vi "File Run.vi"(7 "Write Period":u32=3000, 8 "Error In":errorcluster) -> (0 "Error Out":errorcluster)   [LabVIEW 2017, in "Logger.lvlib"]
doc: "Continuously writes logging statements to the default log file. This VI is called by the File State VI in the background, but if background operation is disabled, then this VI needs to be explicitly placed in the block diagram of the top level application VI."
uses:
  Logger.lvlib
  Private/Control Action.ctl
  Private/File/Action.ctl
  Private/File/File.lvlib
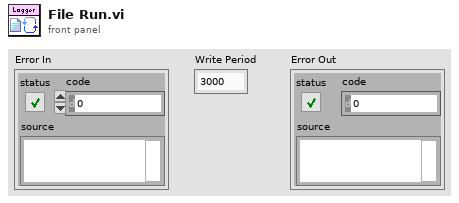
[diagram p1: front panel]
types:
  T1 = typedef "Logger.lvlib/Control Action.ctl" = enum16{"Initialize", "Get", "Set", "Shutdown"}
  T2 = typedef "Logger.lvlib/File.lvlib/Action.ctl" = enum16{"Initialize", "Set Maximum File Size", "Set Maximum File Count", "Set Root Folder", "Set Enable Calendar Folder Tree", "Set File Extension", "Start", "Write", "Stop", "Shutdown"}
  T3 = typedef "Logger.lvlib/Statement.ctl" = cluster{"Time Stamp":timestamp, "Tag":T4, "Source":string, "Message":string}
  T4 = typedef "Logger.lvlib/Tag.ctl" = enum16{"Fatal", "Error", "Warn", "Info", "Debug", "Trace"}
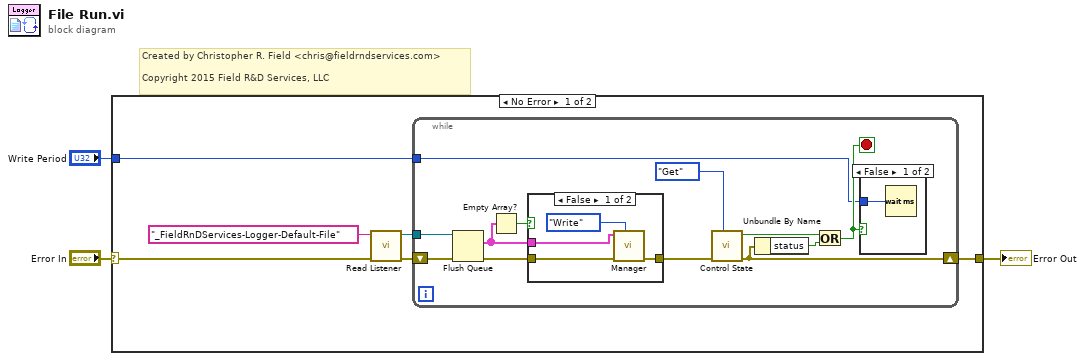
[diagram p0: block diagram]
diagram:
  # "Created by Christopher R. Field <chris@fieldrndservices.com>\n\nCopyright 2015 Field R&D Services, LLC"
  n1 = case shown="No Error" "Error In" {
    selector: "Error In" -> [w9 w28]
    tunnel: [w6 w28] -> w2
    tunnel: "Write Period" -> [w4 _]
    frame No Error {
      n2 = call "Read Listener.vi"("Error In"=w9, "Listener ID"="_FieldRnDServices-Logger-Default-File") -> ("Error Out"=w7:errorcluster, "Listener"=w8:refnum<queue>)  [unwired: 8 in]
      n3 = while {
        tunnel: w8 -> [w21]
        shift-right: [w11] -> w6
        shift-left: w7 -> [w20]
        tunnel: w4 -> [w10]
        stop <- w12 stop-if-true
        n4 = Flush Queue(queue=w21, error in (no error)=w20) -> (remaining elements=w14:T3[], error out=w19:errorcluster)  [unwired: 1 out]
        n5 = Empty Array?(array=w14) -> (empty?=w13:bool)
        n6 = case shown="False" w13 {
          tunnel: w14 -> [w26 _]
          tunnel: w19 -> [w25 w27]
          tunnel: [w23 w27] -> w18
          frame False {
            n7 = call "Manager.vi"("Action"=Action."Write", "Error In"=w25, "Set Value"=w26) -> ("Error Out"=w23:errorcluster)  [unwired: 8 in]
          }
          frame True {
          }
        }
        n8 = call "Control State.vi"("Action"=Control_Action."Get", "Error In"=w18) -> ("Error Out"=w11:errorcluster, "Stop?"=w15:bool)  [unwired: 8 in]
        n9 = Unbundle By Name(w11) -> ("status"=w16:bool)
        n10 = Or(x=w15, y=w16) -> (x .or. y?=w12:bool)
        n11 = case shown="False" w12 {
          tunnel: w10 -> [w22 _]
          frame False {
            n12 = Wait (ms)(milliseconds to wait=w22) -> ()  [unwired: 1 out]
          }
          frame True {
          }
        }
      }
    }
    frame Error {
    }
  }
  "Error Out" <- w2
